vi "Get mean.vi"(10 "Numeric":i32, 11 "file path (dialog if empty)":path) -> (3 "Array":dbl[](array[numeric]))   [LabVIEW 2011]
uses:
  <vilib>/Utility/file.llb/Read From Spreadsheet File (DBL).vi
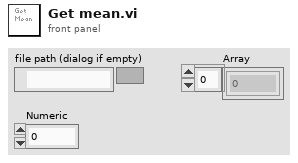
[diagram p1: front panel]
types:
  T1 = typedef "NI_Matrix.lvlib/RealMatrix.ctl" = dbl[][]
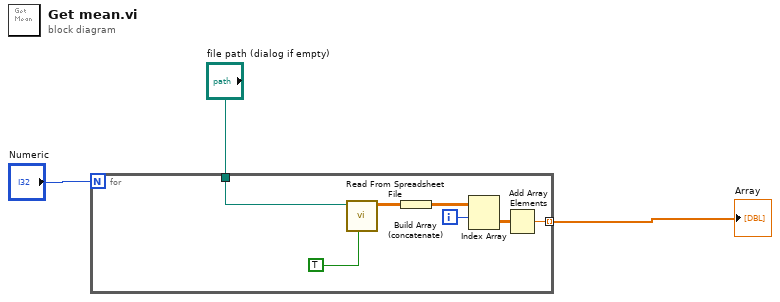
[diagram p0: block diagram]
diagram:
  n1 = for {
    N: "Numeric" -> [_]
    tunnel: [w7] -> w2 mode=indexing
    tunnel: "file path (dialog if empty)" -> [w4]
    i -> [w6]
    n2 = call-poly <vilib>:"Read From Spreadsheet File.vi"("transpose (no:F)"=TRUE, "file path (dialog if empty)"=w4) -> ("all rows"=w9:dbl[][])  [unwired: 5 in, 4 out]
    n3 = Build Array (concatenate)(w9) -> (w5:T1)
    n4 = Index Array(array=w5, index (row)=w6) -> (element=w8:T1)  [unwired: 1 in]
    n5 = Add Array Elements(numeric array=w8) -> (sum=w7:dbl)
  }
  "Array" <- w2
